vi "Register gRPC Methods.vi"(8 "error in (no error)":errorcluster, 11 "Template Server in":refnum<class "ctet_dmm.lvclass">) -> (0 "error out":errorcluster, 3 "Template Server out":refnum<class "ctet_dmm.lvclass">)   [LabVIEW 2019, in "ctet_dmm.lvlib" / "ctet_dmm.lvclass"]
uses:
  ctet_dmm.lvclass
  typeDefs/Server Internal UEs.ctl
  typeDefs/Server Internal Message.ctl
  typeDefs/Server gRPC UEs.ctl
  gRPC lvSupport/Server API/typeDefs/gRPCId Cluster.ctl
  gRPC lvSupport/Server API/typeDefs/grpcId.ctl
  ctet_dmm.lvclass/ctet_dmm.ctl
  gRPC lvSupport/gprc-lvsupport.lvlib
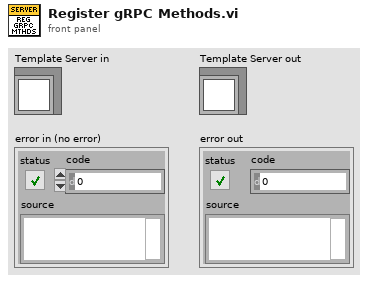
[diagram p1: front panel]
types:
  T1 = typedef "ctet_dmm.lvlib/ctet_dmm.lvclass/Server gRPC UEs.ctl" = cluster{"Invoke gRPC UE":refnum<user-event>, "Query gRPC UE":refnum<user-event>, "Register gRPC UE":refnum<user-event>, "OpenDMMSession gRPC UE":refnum<user-event>, "ConfigureDMM gRPC UE":refnum<user-event>, "PerformDMMMeasurement gRPC UE":refnum<user-event>, "CloseDMMSession gRPC UE":refnum<user-event>, "SelfCalibrateDMM gRPC UE":refnum<user-event>, "ResetDMM gRPC UE":refnum<user-event>, "GetDMMLastExtCalInfo gRPC UE":refnum<user-event>, "GetDMMLastSelfCalInfo gRPC UE":refnum<user-event>}
  T2 = typedef "ctet_dmm.lvlib/ctet_dmm.lvclass/Server Internal UEs.ctl" = cluster{"Invoke Internal UE":refnum<user-event>, "Query Internal UE":refnum<user-event>, "Register Internal UE":refnum<user-event>, "OpenDMMSession Internal UE":refnum<user-event>, "ConfigureDMM Internal UE":refnum<user-event>, "PerformDMMMeasurement Internal UE":refnum<user-event>, "CloseDMMSession Internal UE":refnum<user-event>, "SelfCalibrateDMM Internal UE":refnum<user-event>, "ResetDMM Internal UE":refnum<user-event>, "GetDMMLastExtCalInfo Internal UE":refnum<user-event>, "GetDMMLastSelfCalInfo Internal UE":refnum<user-event>}
  T3 = typedef "ctet_dmm.lvlib/gprc-lvsupport.lvlib/grpcId.ctl" = u64
  T4 = typedef "ctet_dmm.lvlib/ctet_dmm.lvclass/Server Internal Message UE.ctl" = refnum<user-event>
  T5 = typedef "ctet_dmm.lvlib/gprc-lvsupport.lvlib/gRPCId Cluster UE.ctl" = refnum<user-event>
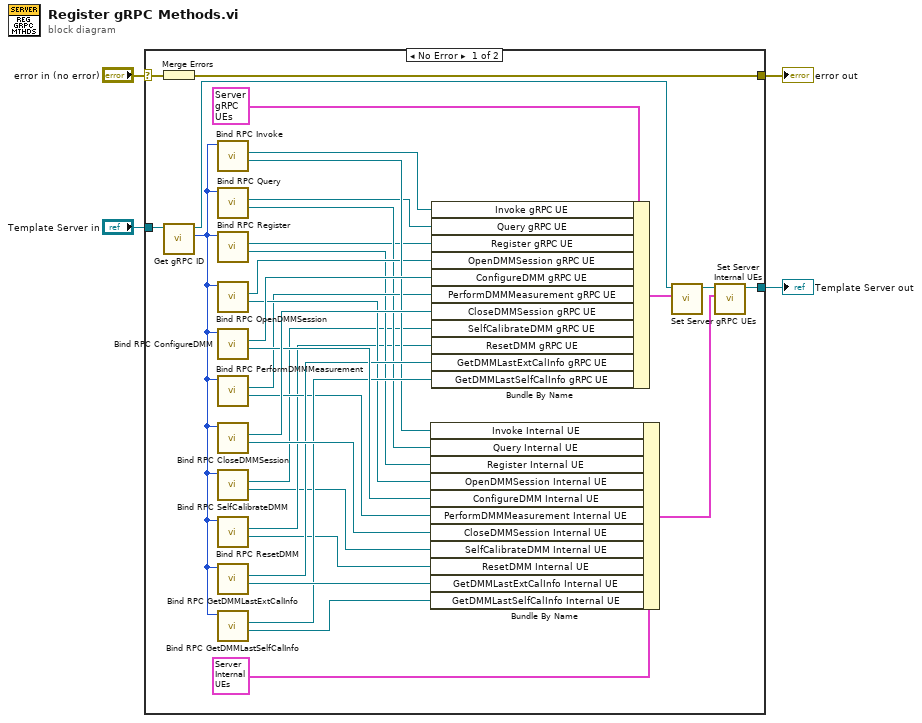
[diagram p0: block diagram]
diagram:
  n1 = case shown="No Error" "error in (no error)" {
    selector: "error in (no error)" -> [w28 w38]
    tunnel: "Template Server in" -> [w36 w39]
    tunnel: [w35 w38] -> w3
    tunnel: [w34 w39] -> w2
    frame No Error {
      n2 = Merge Errors(w28) -> (w35:errorcluster)
      n3 = call "Get gRPC ID.vi"("OOP Server in"=w36) -> ("gRPC ID"=w27:T3, "OOP Server out"=w37:refnum<class "ctet_dmm.lvclass">)  [unwired: 9 in]
      n4 = call "Bind RPC Invoke.vi"("gRPCid server in"=w27) -> ("Invoke Internal UE"=w18:T4, "Invoke gRPC UE"=w17:T5)  [unwired: 7 in, 2 out]
      n5 = call "Bind RPC Query.vi"("gRPCid server in"=w27) -> ("Query Internal UE"=w12:T4, "Query gRPC UE"=w11:T5)  [unwired: 7 in, 2 out]
      n6 = call "Bind RPC Register.vi"("gRPCid server in"=w27) -> ("Register Internal UE"=w10:T4, "Register gRPC UE"=w9:T5)  [unwired: 7 in, 2 out]
      n7 = call "Bind RPC OpenDMMSession.vi"("gRPCid server in"=w27) -> ("OpenDMMSession Internal UE"=w16:T4, "OpenDMMSession gRPC UE"=w15:T5)  [unwired: 7 in, 2 out]
      n8 = call "Bind RPC ConfigureDMM.vi"("gRPCid server in"=w27) -> ("ConfigureDMM Internal UE"=w24:T4, "ConfigureDMM gRPC UE"=w23:T5)  [unwired: 7 in, 2 out]
      n9 = call "Bind RPC PerformDMMMeasurement.vi"("gRPCid server in"=w27) -> ("PerformDMMMeasurement Internal UE"=w14:T4, "PerformDMMMeasurement gRPC UE"=w13:T5)  [unwired: 7 in, 2 out]
      n10 = call "Bind RPC CloseDMMSession.vi"("gRPCid server in"=w27) -> ("CloseDMMSession Internal UE"=w26:T4, "CloseDMMSession gRPC UE"=w25:T5)  [unwired: 7 in, 2 out]
      n11 = call "Bind RPC SelfCalibrateDMM.vi"("gRPCid server in"=w27) -> ("SelfCalibrateDMM Internal UE"=w6:T4, "SelfCalibrateDMM gRPC UE"=w5:T5)  [unwired: 7 in, 2 out]
      n12 = call "Bind RPC ResetDMM.vi"("gRPCid server in"=w27) -> ("ResetDMM Internal UE"=w8:T4, "ResetDMM gRPC UE"=w7:T5)  [unwired: 7 in, 2 out]
      n13 = call "Bind RPC GetDMMLastExtCalInfo.vi"("gRPCid server in"=w27) -> ("GetDMMLastExtCalInfo Internal UE"=w22:T4, "GetDMMLastExtCalInfo gRPC UE"=w21:T5)  [unwired: 7 in, 2 out]
      n14 = call "Bind RPC GetDMMLastSelfCalInfo.vi"("gRPCid server in"=w27) -> ("GetDMMLastSelfCalInfo Internal UE"=w20:T4, "GetDMMLastSelfCalInfo gRPC UE"=w19:T5)  [unwired: 7 in, 2 out]
      n15 = Bundle By Name ("Bundle Internal UEs")(cluster=T2 {"Invoke Internal UE"=refnum, "Query Internal UE"=refnum, "Register Internal UE"=refnum, "OpenDMMSession Internal UE"=refnum, "ConfigureDMM Internal UE"=refnum, "PerformDMMMeasurement Internal UE"=refnum, "CloseDMMSession Internal UE"=refnum, "SelfCalibrateDMM Internal UE"=refnum, "ResetDMM Internal UE"=refnum, "GetDMMLastExtCalInfo Internal UE"=refnum, "GetDMMLastSelfCalInfo Internal UE"=refnum} ("Server Internal UEs"), "Invoke Internal UE"=w18, "Query Internal UE"=w12, "Register Internal UE"=w10, "OpenDMMSession Internal UE"=w16, "ConfigureDMM Internal UE"=w24, "PerformDMMMeasurement Internal UE"=w14, "CloseDMMSession Internal UE"=w26, "SelfCalibrateDMM Internal UE"=w6, "ResetDMM Internal UE"=w8, "GetDMMLastExtCalInfo Internal UE"=w22, "GetDMMLastSelfCalInfo Internal UE"=w20) -> (w33:T2)
      n16 = Bundle By Name ("Bundle gRPC UEs")(cluster=T1 {"Invoke gRPC UE"=refnum, "Query gRPC UE"=refnum, "Register gRPC UE"=refnum, "OpenDMMSession gRPC UE"=refnum, "ConfigureDMM gRPC UE"=refnum, "PerformDMMMeasurement gRPC UE"=refnum, "CloseDMMSession gRPC UE"=refnum, "SelfCalibrateDMM gRPC UE"=refnum, "ResetDMM gRPC UE"=refnum, "GetDMMLastExtCalInfo gRPC UE"=refnum, "GetDMMLastSelfCalInfo gRPC UE"=refnum} ("gRPC Server Method Events"), "Invoke gRPC UE"=w17, "Query gRPC UE"=w11, "Register gRPC UE"=w9, "OpenDMMSession gRPC UE"=w15, "ConfigureDMM gRPC UE"=w23, "PerformDMMMeasurement gRPC UE"=w13, "CloseDMMSession gRPC UE"=w25, "SelfCalibrateDMM gRPC UE"=w5, "ResetDMM gRPC UE"=w7, "GetDMMLastExtCalInfo gRPC UE"=w21, "GetDMMLastSelfCalInfo gRPC UE"=w19) -> (w30:T1)
      n17 = call "Set Server gRPC UEs.vi"("Server gRPC UEs"=w30, "OOP Server in"=w37) -> ("OOP Server out"=w31:refnum<class "ctet_dmm.lvclass">)  [unwired: 9 in]
      n18 = call "Set Server Internal UEs.vi"("Server Internal UEs"=w33, "OOP Server in"=w31) -> ("OOP Server out"=w34:refnum<class "ctet_dmm.lvclass">)  [unwired: 9 in]
    }
    frame Error {
    }
  }
  "error out" <- w3
  "Template Server out" <- w2
